vi "Sensor Interface View.vi"(8 "error in (no error)":errorcluster, 11 "View Model":T1) -> (0 "error out":errorcluster)   [LabVIEW 2017]
doc: "The interface where a user simulates the depositing of checks or cash and the dispensing of cash.\n[Covers: UI4]"
uses:
  View Model/Controls/View Model.ctl
  View Model/Controls/Shared Model.ctl
  Error Handler/Controls/Error Model.ctl
  Error Handler/Controls/Error Data.ctl
  Error Handler/Controls/Error Type.ctl
  Error Handler/Controls/Error Source.ctl
  Configuration/Controls/Config Model.ctl
  Configuration/Controls/Config CMD.ctl
  Configuration/Controls/Config Command.ctl
  Controller/Controls/Controller Model.ctl
  Controller/Controls/Controller Overhead.ctl
panel:
  in  "Fund Dispensed":bool
  in  "Deposit Received":bool
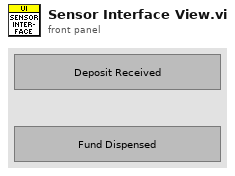
[diagram p1: front panel]
types:
  T1 = typedef "View Model.ctl" = cluster{"Shared Model":T2, "Error Model":T3, "Config Model":T4, "Controller Model":T5}
  T2 = typedef "Shared Model.ctl" = cluster{"Stop":refnum<user-event>, "Stop DVR":refnum<data-value>}
  T3 = typedef "Error Model.ctl" = cluster{"Error":refnum<user-event>}
  T4 = typedef "Config Model.ctl" = cluster{"Config CMD":refnum<user-event>}
  T5 = typedef "Controller Model.ctl" = cluster{"Deposit Received":refnum<user-event>, "Funds Dispensed":refnum<user-event>, "Overhead DVR":refnum<data-value>}
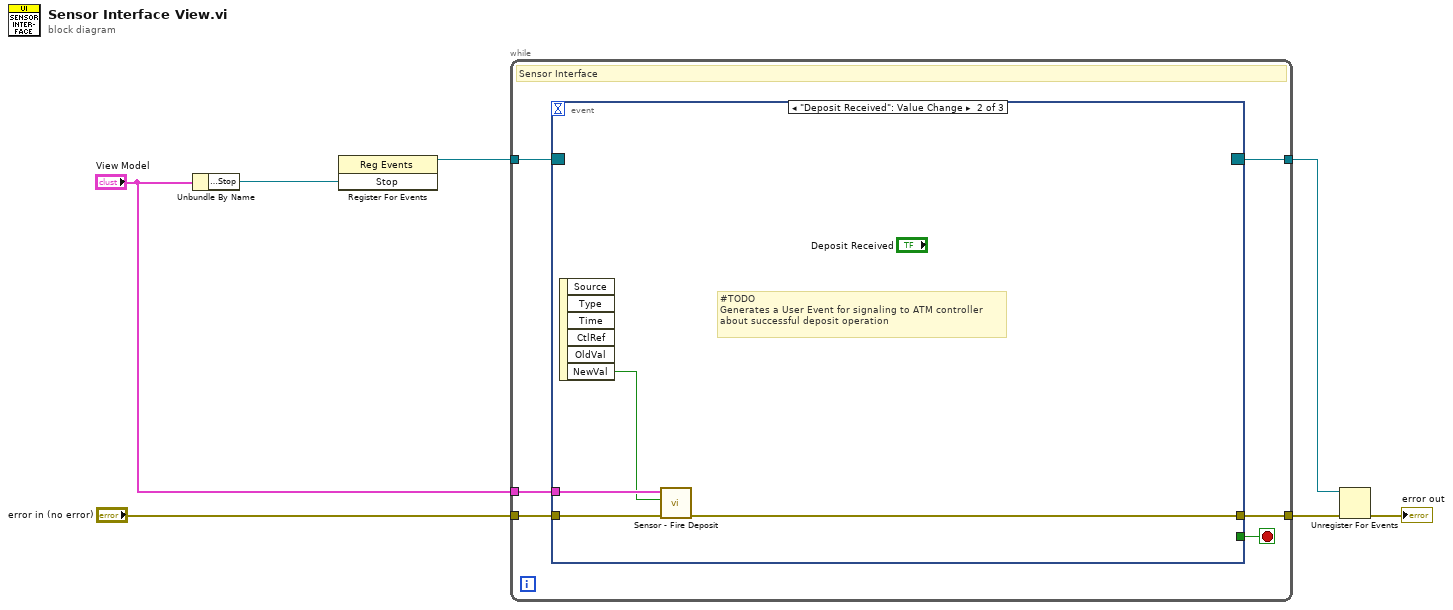
[diagram p0: block diagram]
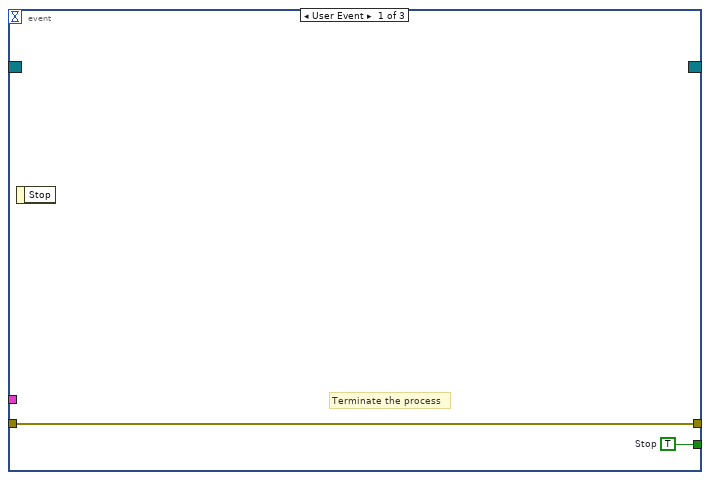
[diagram p2: hidden frame]
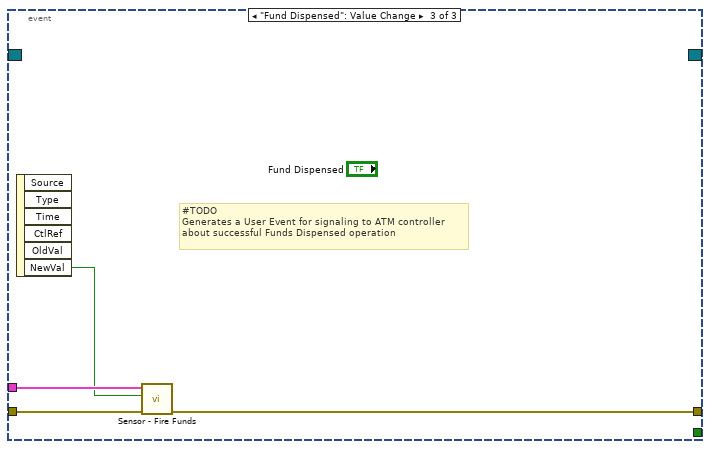
[diagram p3: hidden frame]
diagram:
  n1 = Unbundle By Name("View Model") -> ("Shared Model.Stop"=w7:refnum<user-event>)
  n2 = register-events(w7) -> (reference out=w6:refnum<event-registration>)  [unwired: 2 in, 1 out]
  n3 = while {
    tunnel: w6 -> [w13]
    tunnel: [w12] -> w5
    tunnel: "error in (no error)" -> [w11]
    tunnel: [w10] -> w2
    tunnel: "View Model" -> [w8]
    stop <- w9 stop-if-true
    # "Sensor Interface"
    n4 = event shown="[1] \"Deposit Received\": Value Change" {
      selector: w13 -> [_ _ _]
      dyn-events: [_ _ _] -> w12
      timeout: _ -> [_ _ _]
      tunnel: w11 -> [w15 w19 w23]
      tunnel: [w15 w16 w20] -> w10
      tunnel: [w14 _ _] -> w9
      tunnel: w8 -> [_ w18 w22]
      event User Event {
        w14 = TRUE  # Stop
        # "Terminate the process"
        n5 = event-data() -> ()  [unwired: 1 in, 1 out]
      }
      event "Deposit Received": Value Change {
        # "#TODO\nGenerates a User Event for signaling to ATM controller\nabout successful deposit operation"
        n6 = event-data() -> ("NewVal"=w17:bool)  [unwired: 1 in, 5 out]
        n7 = call "Sensor - Fire Deposit.vi"("error in (no error)"=w19, "Deposit Received"=w17, "View Model"=w18) -> ("error out"=w16:errorcluster)  [unwired: 7 in, 1 out]
      }
      event "Fund Dispensed": Value Change {
        # "#TODO\nGenerates a User Event for signaling to ATM controller\nabout successful Funds Dispensed operation"
        n8 = event-data() -> ("NewVal"=w21:bool)  [unwired: 1 in, 5 out]
        n9 = call "Sensor - Fire Funds.vi"("error in (no error)"=w23, "Funds Dispensed"=w21, "View Model"=w22) -> ("error out"=w20:errorcluster)  [unwired: 7 in, 1 out]
      }
    }
  }
  n10 = Unregister For Events(event registration refnum=w5, error in=w2) -> (error out=→"error out":errorcluster)
